vi "Pulse.vi"(2 "Miliseconds to Wait for Pulse":u32=1000, 3 "Reverse Button":bool, 4 "Pulse Button":bool, 5 "Forward Button":bool) -> (0 "Motor2 Output":dbl, 1 "Motor1 Output":dbl)   [LabVIEW 2017]
panel:
  # "Takes three Boolean Inputs (seen above):\nPulse has #1 priority, then Reverse, then Forward.\nIf Pulse is pressed, invert motors for one second. Continue to \npress Pulse for longer invert. Forward and reverse are self explanatory\nTwo integer outputs are intended for motor control.\nMs to Wait input impacts the amount of time that the motors pulse. E.g.\n1000 is one second of pulse."
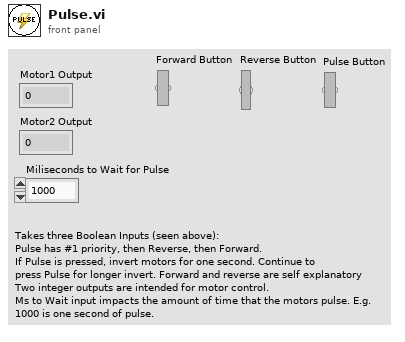
[diagram p1: front panel]
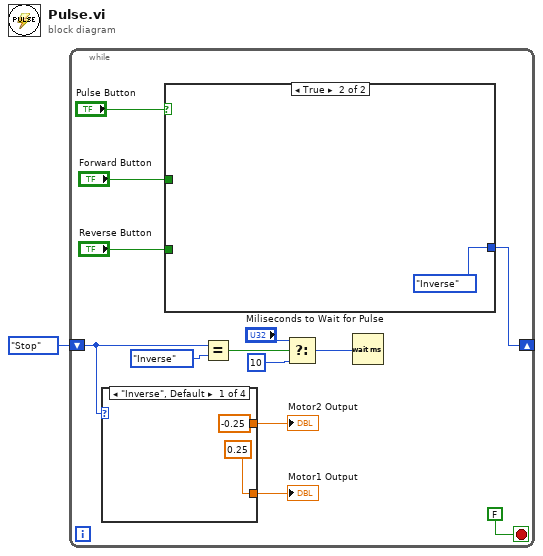
[diagram p0: block diagram]
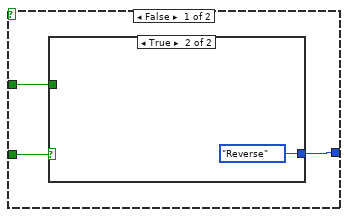
[diagram p2: hidden frame]
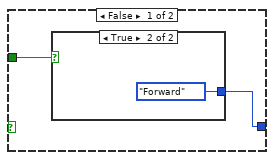
[diagram p3: hidden frame]
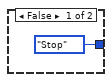
[diagram p4: hidden frame]
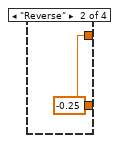
[diagram p5: hidden frame]
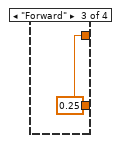
[diagram p6: hidden frame]
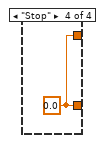
[diagram p7: hidden frame]
diagram:
  n1 = while {
    shift-right: [w8] -> _
    shift-left: enum16{"Stop", "Inverse", "Reverse", "Forward"}."Stop" ("State!") -> [w7]
    stop <- FALSE stop-if-true
    n2 = case shown="\"Inverse\", Default" w7 {
      tunnel: [0.25 w26 w27 w28] -> w14
      tunnel: [-0.25 w26 w27 w28] -> w13
      frame "Inverse", Default {
      }
      frame "Reverse" {
        w26 = -0.25
      }
      frame "Forward" {
        w27 = 0.25
      }
      frame "Stop" {
        w28 = 0.0
      }
    }
    "Motor1 Output" <- w14
    "Motor2 Output" <- w13
    n3 = case shown="True" "Pulse Button" {
      tunnel: "Reverse Button" -> [w17 _]
      tunnel: "Forward Button" -> [w16 _]
      tunnel: [w15 enum16{"Stop", "Inverse", "Reverse", "Forward"}."Inverse" ("State!")] -> w8
      frame False {
        n4 = case shown="True" w17 {
          tunnel: w16 -> [w19 _]
          tunnel: [w18 enum16{"Stop", "Inverse", "Reverse", "Forward"}."Reverse" ("State!")] -> w15
          frame False {
            n5 = case shown="True" w19 {
              tunnel: [enum16{"Stop", "Inverse", "Reverse", "Forward"}."Stop" ("State!") enum16{"Stop", "Inverse", "Reverse", "Forward"}."Forward" ("State!")] -> w18
              frame False {
              }
              frame True {
              }
            }
          }
          frame True {
          }
        }
      }
      frame True {
      }
    }
    n6 = Equal?(x=w7, y=enum16{"Stop", "Inverse", "Reverse", "Forward"}."Inverse") -> (x = y?=w5:bool)
    n7 = Select(t="Miliseconds to Wait for Pulse", s=w5, f=u32 10 ("milliseconds to wait")) -> (s? t:f=w3:u32)
    n8 = Wait (ms)(milliseconds to wait=w3) -> ()  [unwired: 1 out]
  }
